vi "Get Local and ECAT Refs.vi"(8 "error in (no error)":errorcluster, 11 "Device Reference in":T1 format="%.0x") -> (0 "error out":errorcluster, 2 "ECAT Master Refs":T1[](array[typedef]) format="%.0x", 3 "Local Chassis Refs":T1[](array[typedef]) format="%.0x")   [LabVIEW 2019, in "SEECD Engine.lvlib"]
uses:
  SEECD Engine.lvlib
  <vilib>/NI VeriStand/Custom Device API/Custom Device Item Ref.ctl
  Shared/Globals/Scan Engine GUIDs.vi
  <vilib>/NI VeriStand/Custom Device API/Custom Device API.lvlib
  Shared/SEECD Shared.lvlib
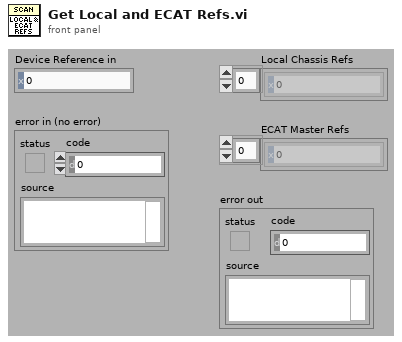
[diagram p1: front panel]
types:
  T1 = typedef "Custom Device API.lvlib/Custom Device Item Ref.ctl" = u64
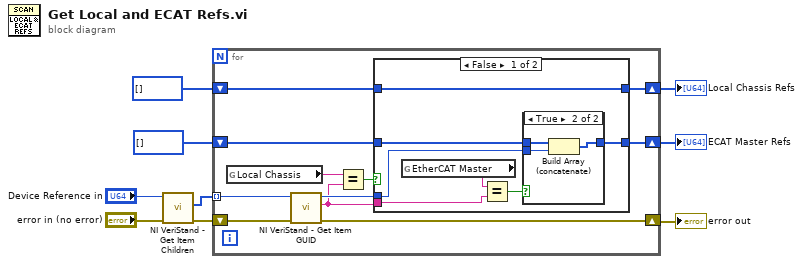
[diagram p0: block diagram]
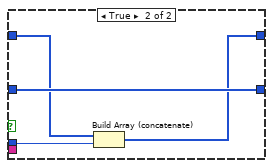
[diagram p3: hidden frame]
diagram:
  n1 = call <vilib>:"NI VeriStand - Get Item Children.vi"("error in (no error)"="error in (no error)", "Item Ref in"="Device Reference in") -> ("error out"=w4:errorcluster, "Child Refs"=w2:T1[])  [unwired: 6 in, 2 out]
  n2 = for {
    tunnel: w2 -> [w20] mode=indexing
    shift-right: [w13] -> w9
    shift-left: T1[] [] -> [w16]
    shift-right: [w14] -> w6
    shift-left: T1[] [] -> [w15]
    shift-right: [w10] -> w7
    shift-left: w4 -> [w11]
    n3 = global read "Scan Engine GUIDs.vi" "Local Chassis"() -> (w19:string)
    n4 = call <vilib>:"NI VeriStand - Get Item GUID.vi"("error in (no error)"=w11, "Item Ref in"=w20) -> ("error out"=w10:errorcluster, "GUID"=w12:string, "Item Ref out"=w18:T1)  [unwired: 7 in]
    n5 = Equal?(x=w19, y=w12) -> (x = y?=w17:bool)
    n6 = case shown="False" w17 {
      tunnel: w18 -> [w22 w33]
      tunnel: w16 -> [w23 w35]
      tunnel: w15 -> [w25 w34]
      tunnel: [w25 w32] -> w14
      tunnel: [w21 w35] -> w13
      tunnel: w12 -> [w26 _]
      frame False {
        n7 = global read "Scan Engine GUIDs.vi" "EtherCAT Master"() -> (w27:string)
        n8 = Equal?(x=w27, y=w26) -> (x = y?=w24:bool)
        n9 = case shown="True" w24 {
          tunnel: w23 -> [w28 w31]
          tunnel: w22 -> [_ w30]
          tunnel: [w28 w29] -> w21
          frame False {
          }
          frame True {
            n10 = Build Array (concatenate)(w31, w30) -> (w29:T1[])
          }
        }
      }
      frame True {
        n11 = Build Array (concatenate)(w34, w33) -> (w32:T1[])
      }
    }
  }
  "ECAT Master Refs" <- w9
  "error out" <- w7
  "Local Chassis Refs" <- w6
